vi "Main Controls Systemv9.vi"() -> ()   [LabVIEW 2021]
uses:
  Main Controls System v8.0/AutoAge Globals.vi
  Main Control Globals.vi
panel:
  in  "Clear Data":bool
  out "Functional  Data":string
  in  "Run Functional Test":bool
  in  "View Warm-up":bool
  in  "Exit":bool
  in  "System #":u8=1 min=1 max=4 step=3
  in  "Aging Summary":bool
  in  "Add Units":bool
  in  "Remove Units":bool
  in  "Xref Osc":bool
  in  "List Positions":bool
  in  "Display Rack Summary":bool
  # "Automated Ageing System - Analysis and Scheduler"
  # "Analysis Functions"
  # "Scheduler Functions"
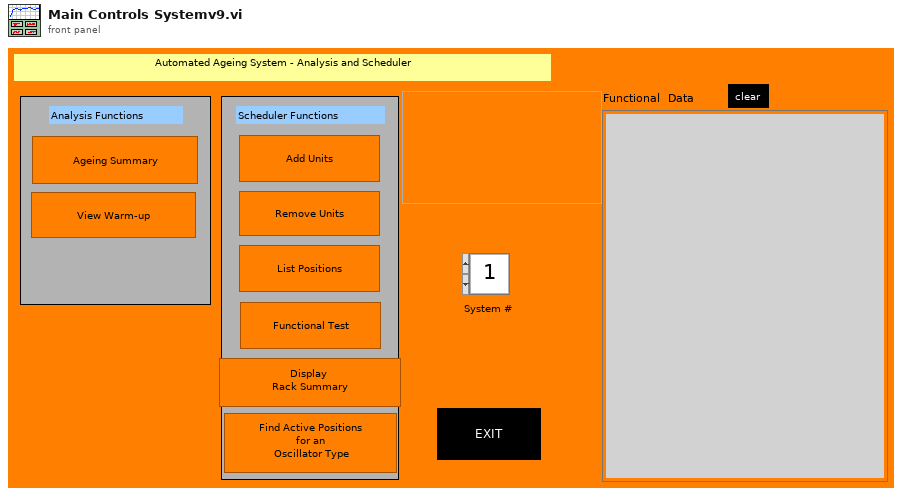
[diagram p1: front panel]
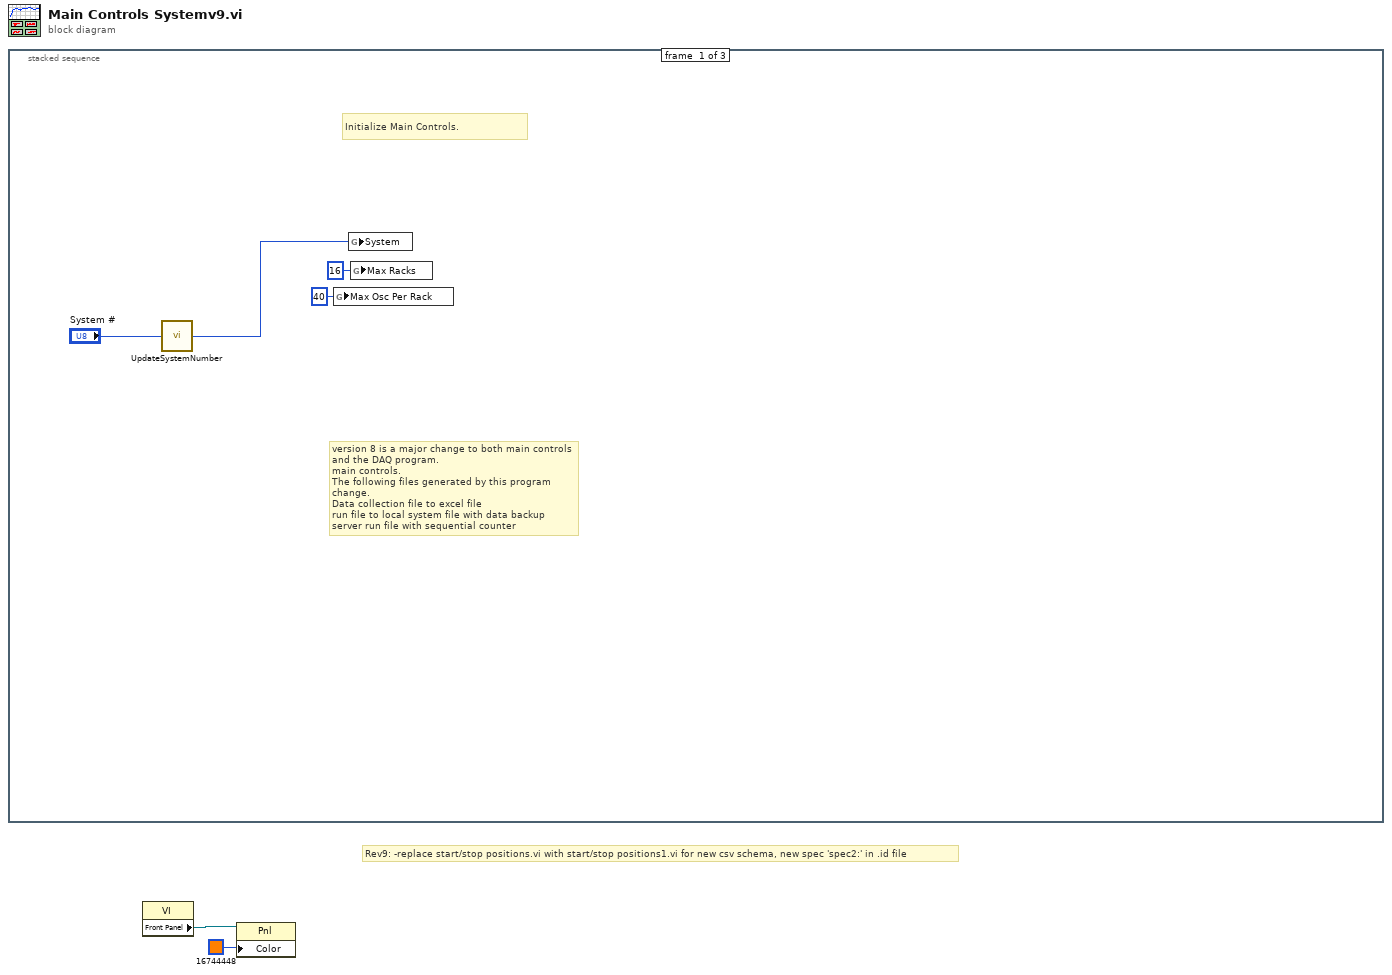
[diagram p0: block diagram]
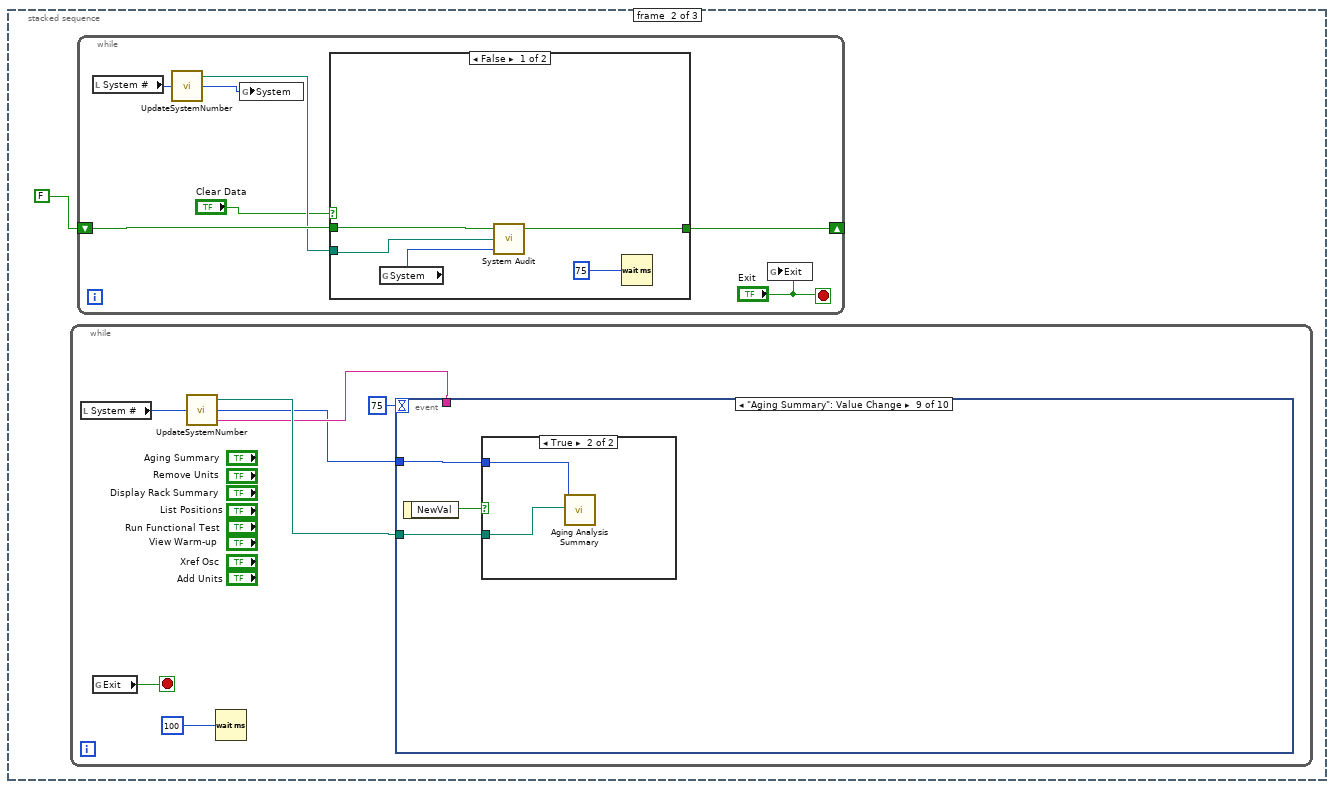
[diagram p2: hidden frame]
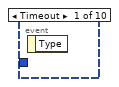
[diagram p3: hidden frame]
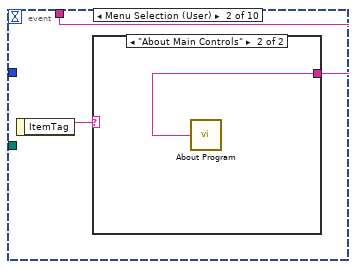
[diagram p4: hidden frame]
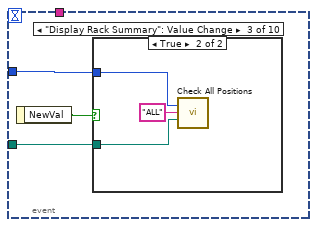
[diagram p6: hidden frame]
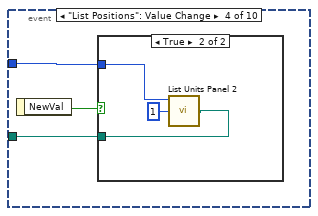
[diagram p8: hidden frame]
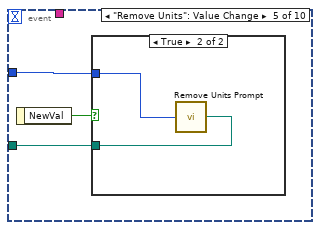
[diagram p10: hidden frame]
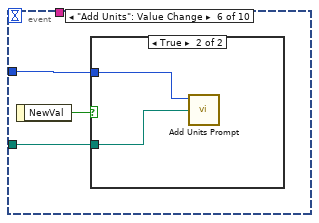
[diagram p12: hidden frame]
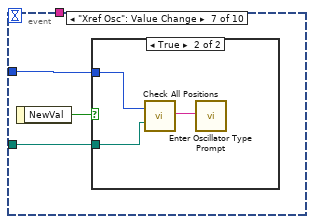
[diagram p14: hidden frame]
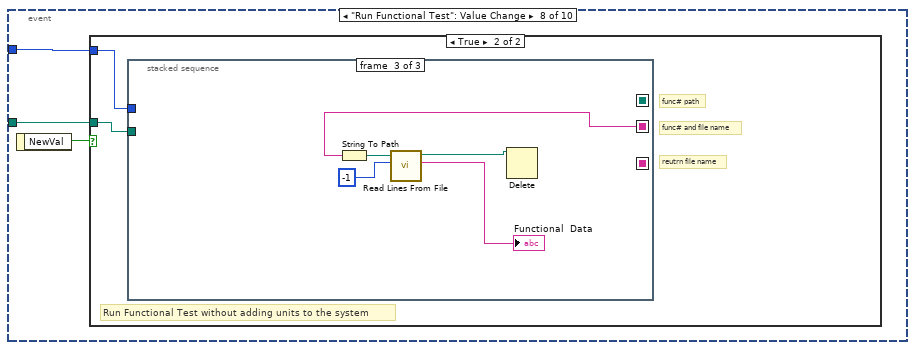
[diagram p16: hidden frame]
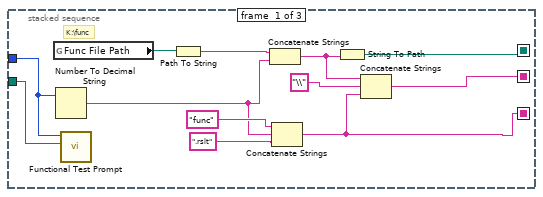
[diagram p18: hidden frame]
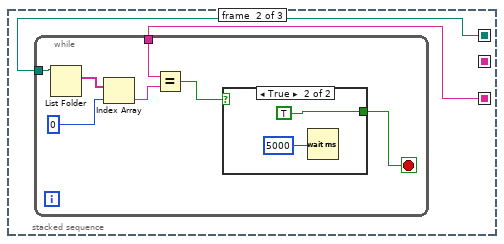
[diagram p19: hidden frame]
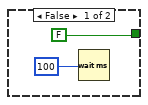
[diagram p20: hidden frame]
diagram:
  # "Rev9: -replace start/stop positions.vi with start/stop positions1.vi for new csv schema, new spec 'spec2:' in .id file"
  n1 = stacked-sequence {
    frame #0 {
      # "version 8 is a major change to both main controls and the DAQ program. \nmain controls.\nThe following files generated by this program change.\nData collection file to excel file\nrun file to local system file with data backup\nserver run file with sequential counter"
      # "Initialize Main Controls."
      n2 = call "UpdateSystemNumber.vi"("InSystemNo"="System #") -> ("SystemNo"=w3:i8)  [unwired: 2 out]
      n3 = global write "AutoAge Globals.vi" "Max Osc Per Rack"(u16 40 ("Max Osc Per Rack")) -> ()
      n4 = global write "AutoAge Globals.vi" "System"(w3) -> ()
      n5 = global write "AutoAge Globals.vi" "Max Racks"(u8 16 ("Max Racks")) -> ()
    }
    frame #1 {
      n6 = while {
        stop <- w14 stop-if-true
        n7 = local read "System #"() -> (w11:u8)
        n8 = global read "Main Control Globals.vi" "Exit"() -> (w14:bool)
        n9 = call "UpdateSystemNumber.vi"("InSystemNo"=w11) -> ("ConfigPath"=w10:path, "SystemNo"=w8:i8, "Title Block"=w9:string)
        n10 = Wait (ms)(milliseconds to wait=u32 100) -> ()  [unwired: 1 out]
        n11 = event shown="[8] \"Aging Summary\": Value Change" {
          selector: _ -> [_ _ _ _ _ _ _ _ _ _]
          dyn-events: _ -> [_ _ _ _ _ _ _ _ _ _]
          timeout: 75 -> [_ _ _ _ _ _ _ _ _ _]
          tunnel: w8 -> [_ _ w19 w25 w31 w36 w41 w47 w82 w86]
          tunnel: w10 -> [_ _ w18 w24 w30 w35 w40 w46 w81 _]
          tunnel: w9 -> [_ w15 _ _ _ _ _ _ _ _]
          event Timeout {
            n12 = event-data() -> ()  [unwired: 1 in, 1 out]
          }
          event Menu Selection (User) {
            n13 = event-data() -> ("ItemTag"=w16:string)  [unwired: 1 in]
            n14 = case shown="\"About Main Controls\"" w16 {
              tunnel: w15 -> [_ w17]
              frame "False", Default {
              }
              frame "About Main Controls" {
                n15 = call "About Program.vi"("Diplay Text In"=w17) -> ()  [unwired: 1 in]
              }
            }
          }
          event "Display Rack Summary": Value Change {
            n16 = event-data() -> ("NewVal"=w20:bool)  [unwired: 1 in]
            n17 = case shown="True" w20 {
              tunnel: w19 -> [_ w21]
              tunnel: w18 -> [_ w22]
              frame False {
              }
              frame True {
                n18 = call "Check All Positions"("Oscillator Type"="ALL", "AutoAge.ini  File Path"=w22, "Sytem #"=w21) -> ()  [unwired: 1 in]
              }
            }
          }
          event "List Positions": Value Change {
            n19 = event-data() -> ("NewVal"=w26:bool)  [unwired: 1 in]
            n20 = case shown="True" w26 {
              tunnel: w25 -> [_ w29]
              tunnel: w24 -> [_ w28]
              frame False {
              }
              frame True {
                n21 = call "List Units Panel 2.vi"("System#"=w29, "Rack Number"=i8 1, "AutoAge.ini  File Path"=w28) -> ()  [unwired: 13 in]
              }
            }
          }
          event "Remove Units": Value Change {
            n22 = event-data() -> ("NewVal"=w32:bool)  [unwired: 1 in]
            n23 = case shown="True" w32 {
              tunnel: w31 -> [_ w34]
              tunnel: w30 -> [_ w33]
              frame False {
              }
              frame True {
                n24 = call "Remove Units Prompt"("AutoAge.ini  File Path"=w33, "System #"=w34) -> ()
              }
            }
          }
          event "Add Units": Value Change {
            n25 = event-data() -> ("NewVal"=w37:bool)  [unwired: 1 in]
            n26 = case shown="True" w37 {
              tunnel: w36 -> [_ w39]
              tunnel: w35 -> [_ w38]
              frame False {
              }
              frame True {
                n27 = call "Add Units Prompt"("AutoAge.ini  File Path"=w38, "System#"=w39) -> ()  [unwired: 10 in]
              }
            }
          }
          event "Xref Osc": Value Change {
            n28 = event-data() -> ("NewVal"=w42:bool)  [unwired: 1 in]
            n29 = case shown="True" w42 {
              tunnel: w41 -> [_ w44]
              tunnel: w40 -> [_ w43]
              frame False {
              }
              frame True {
                n30 = call "Enter Oscillator Type Prompt"() -> ("Osc Type Found"=w45:string)  [unwired: 1 in]
                n31 = call "Check All Positions"("Oscillator Type"=w45, "AutoAge.ini  File Path"=w43, "Sytem #"=w44) -> ()  [unwired: 1 in]
              }
            }
          }
          event "Run Functional Test": Value Change {
            n32 = event-data() -> ("NewVal"=w48:bool)  [unwired: 1 in]
            n33 = case shown="True" w48 {
              tunnel: w47 -> [_ w50]
              tunnel: w46 -> [_ w49]
              frame False {
              }
              frame True {
                # "reutrn file name"
                # "func# and file name"
                # "func# path"
                # "Run Functional Test without adding units to the system"
                n34 = stacked-sequence {
                  seq-local: [w53 _ _] -> [_ _ w77]
                  seq-local: [w59 _ _] -> [_ w64 _]
                  seq-local: [w51 _ _] -> [_ w63 _]
                  tunnel: w50 -> [w62 _ _]
                  tunnel: w49 -> [w61 _ _]
                  frame #0 {
                    # "K:\\func"
                    n35 = global read "AutoAge Globals.vi" "Func File Path"() -> (w60:path)
                    n36 = Number To Decimal String(number=w62) -> (decimal integer string=w56:string)  [unwired: 1 in]
                    n37 = call "Functional Test Prompt.vi"("AutoAge.ini  File Path"=w61, "System#"=w62) -> ()  [unwired: 10 in]
                    n38 = Path To String(path=w60) -> (string=w52:string)
                    n39 = Concatenate Strings(w52, w56) -> (w55:string)
                    n40 = Concatenate Strings("func", w56, ".rslt") -> (w51:string)
                    n41 = String To Path(string=w55) -> (path=w59:path)
                    n42 = Concatenate Strings(w55, "\\", w51) -> (w53:string)
                  }
                  frame #1 {
                    n43 = while {
                      tunnel: w64 -> [w71]
                      tunnel: w63 -> [w65]
                      stop <- w66 stop-if-true
                      n44 = List Folder(path=w71) -> (filenames=w69:string[])  [unwired: 3 in, 3 out]
                      n45 = Index Array(array=w69, index=0) -> (element=w68:string)
                      n46 = Equal?(x=w65, y=w68) -> (x = y?=w67:bool)
                      n47 = case shown="True" w67 {
                        tunnel: [FALSE TRUE] -> w66
                        frame False {
                          n48 = Wait (ms)(milliseconds to wait=100) -> ()  [unwired: 1 out]
                        }
                        frame True {
                          n49 = Wait (ms)(milliseconds to wait=5000) -> ()  [unwired: 1 out]
                        }
                      }
                    }
                  }
                  frame #2 {
                    n50 = String To Path(string=w77) -> (path=w79:path)
                    n51 = call <vilib>:"Read Lines From File.vi"("file path (dialog if empty)"=w79, "number of lines (all:-1)"=-1) -> ("new file path (Not A Path if cancelled)"=w80:path, "line string"=→"Functional  Data":string)  [unwired: 4 in, 2 out]
                    n52 = Delete(path (use dialog)=w80) -> ()  [unwired: 4 in, 3 out]
                  }
                }
              }
            }
          }
          event "Aging Summary": Value Change {
            n53 = event-data() -> ("NewVal"=w83:bool)  [unwired: 1 in]
            n54 = case shown="True" w83 {
              tunnel: w82 -> [_ w85]
              tunnel: w81 -> [_ w84]
              frame False {
              }
              frame True {
                n55 = call "Aging Analysis Summary"("AutoAge.ini  File Path"=w84, "System #"=w85) -> ()  [unwired: 8 in]
              }
            }
          }
          event "View Warm-up": Value Change {
            n56 = event-data() -> ("NewVal"=w87:bool)  [unwired: 1 in]
            n57 = case shown="True" w87 {
              tunnel: w86 -> [_ w90]
              frame False {
              }
              frame True {
                n58 = call "CMF - View Warmer.vi"("Position Number"=i8 1, "Rack"=u8 1, "System"=w90) -> ()
              }
            }
          }
        }
      }
      n59 = while {
        shift-left: FALSE -> [w96]
        shift-right: [w95] -> _
        stop <- "Exit" stop-if-true
        n60 = local read "System #"() -> (w94:u8)
        n61 = call "UpdateSystemNumber.vi"("InSystemNo"=w94) -> ("ConfigPath"=w93:path, "SystemNo"=w92:i8)  [unwired: 1 out]
        n62 = global write "AutoAge Globals.vi" "System"(w92) -> ()
        n63 = case shown="False" "Clear Data" {
          tunnel: w93 -> [w101 _]
          tunnel: w96 -> [w100 w103]
          tunnel: [w99 w103] -> w95
          frame False {
            n64 = global read "AutoAge Globals.vi" "System"() -> (w98:u8)
            n65 = call "System Audit.vi"("Sytem #"=w98, "AutoAge.ini  File Path"=w101, "Status In"=w100) -> ("Status Out"=w99:bool)  [unwired: 2 in]
            n66 = Wait (ms)(milliseconds to wait=u32 75) -> ()  [unwired: 1 out]
          }
          frame True {
            (unwired) ""
          }
        }
        n67 = global write "Main Control Globals.vi" "Exit"("Exit") -> ()
      }
    }
    frame #2 {
      w104 = FALSE
      n68 = local write "Exit"(w104) -> ()
      n69 = global write "Main Control Globals.vi" "Exit"(w104) -> ()
      n70 = Quit LabVIEW(quit? (T)=w104) -> ()
    }
  }
  n71 = property class="VI"() -> ("Front Panel"=w2:refnum<vi>)  [unwired: 2 in, 2 out]
  n72 = property class="Pnl"(reference=w2, "Color"=u32 16744448) -> ()  [unwired: 1 in, 2 out]
